vi "Read Supported Functions.vi"(8 "error in (no error)":errorcluster, 11 "Mag Lab Hardware in":refnum<class "Mag Lab Hardware.lvclass">) -> (0 "error out":errorcluster, 2 "Supported Functions":T1[](array[typedef]), 3 "Mag Lab Hardware out":refnum<class "Mag Lab Hardware.lvclass">)   [LabVIEW 2015, in "Mag Lab Hardware.lvclass"]
uses:
  Mag Lab Hardware.lvclass
  Mag Lab Hardware Function.ctl
  Mag Lab Hardware.lvclass/Mag Lab Hardware.ctl
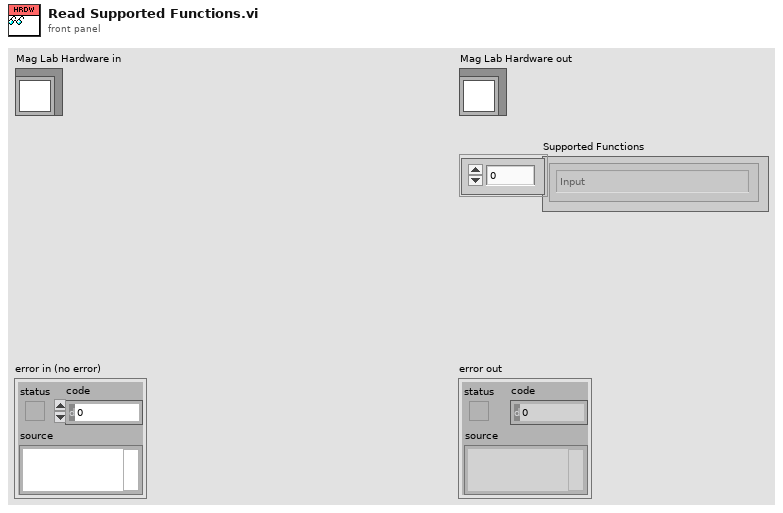
[diagram p1: front panel]
types:
  T1 = typedef "Mag Lab Hardware Function.ctl" = enum16{"Input", "Voltmeter", "Output", "Current source", "Digitizer", "Temperature controller"}
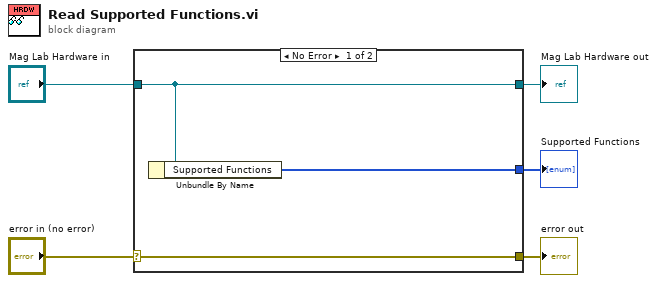
[diagram p0: block diagram]
diagram:
  n1 = case shown="No Error" "error in (no error)" {
    selector: "error in (no error)" -> [w8 w9]
    tunnel: [w8 w9] -> w4
    tunnel: [w7 w10] -> w2
    tunnel: "Mag Lab Hardware in" -> [w7 w10]
    tunnel: [w6 _] -> w1
    frame No Error {
      n2 = Unbundle By Name(w7) -> ("Supported Functions"=w6:T1[])
    }
    frame Error {
    }
  }
  "error out" <- w4
  "Mag Lab Hardware out" <- w2
  "Supported Functions" <- w1
